vi "part2.vi"() -> ()   [LabVIEW 2019]
panel:
  in  "stop":bool
  out "LED":bool
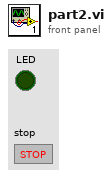
[diagram p1: front panel]
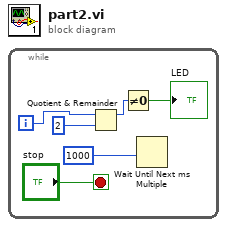
[diagram p0: block diagram]
diagram:
  n1 = while {
    i -> [w2]
    stop <- "stop" stop-if-true
    n2 = Quotient & Remainder(x=w2, y=2) -> (x-y*floor(x/y)=w3:i32)  [unwired: 1 out]
    n3 = Not Equal To 0?(x=w3) -> (x != 0?=→"LED":bool)
    n4 = Wait Until Next ms Multiple(millisecond multiple=1000) -> ()  [unwired: 1 out]
  }
